vi "Send Light Message.vi"(9 "Lights":T1) -> (0 "error out":errorcluster)   [LabVIEW 2016]
uses:
  Light Reference.ctl
  <vilib>/Rock Robotics/WPI/SerialPort/WPI_SerialPortRef.ctl
  LED Send Global.vi
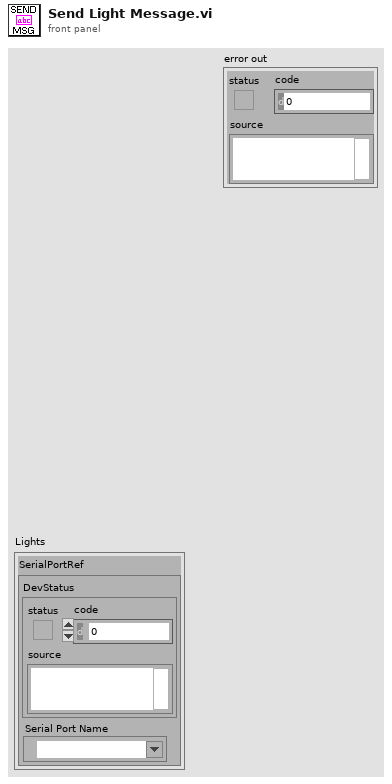
[diagram p1: front panel]
types:
  T1 = typedef "Light Reference.ctl" = cluster{"SerialPortRef":T2}
  T2 = typedef "WPI_SerialPortRef.ctl" = cluster{"DevStatus":errorcluster, "Serial Port Name":refnum<visa-resource-name>}
  T3 = typedef "LED Send Global.ctl" = cluster{"Underglow States":cluster{"RED":bool, "BLUE":bool}, "Hopper States":cluster{"No Shooter Power":bool, "1 RED":bool, "2 RED":bool, "3 RED":bool, "1 YEL 3 RED":bool, "2 YEL 3 RED":bool, "3 YEL 3 RED":bool, "1 GRN 3 YEL 3 RED":bool, "2 GRN 3 YEL 3 RED":bool, "3 GRN 3 YEL 3 RED":bool, "All GRN":bool, "Shooter w/Agitator":bool}, "License Plate States":cluster{"Auton States":cluster{"Do Nothing":bool, "Gear":bool, "Gear & Baseline":bool, "Gear & Shooter":bool, "Shooter":bool, "Shooter & Ball Dump":bool}, "Drive Train":cluster{"High Gear":bool, "Low Gear":bool}}, "Misc":cluster{"Pit/Demo":bool}, "Lights":cluster{"Underglow":string, "License Plate":string, "Hopper":string}}
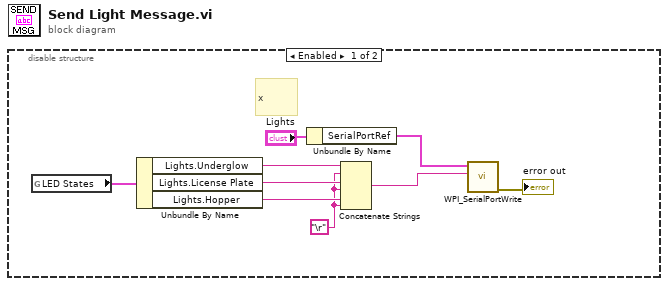
[diagram p0: block diagram]
diagram:
  n1 = disable-structure shown="Enabled" {
    frame Enabled {
      w5 = "\r"
      # "x"
      n2 = global read "LED Send Global.vi" "LED States"() -> (w3:T3)
      n3 = Unbundle By Name(w3) -> ("Lights.Underglow"=w9:string, "Lights.License Plate"=w6:string, "Lights.Hopper"=w7:string)
      n4 = Unbundle By Name("Lights") -> ("SerialPortRef"=w1:T2)
      n5 = Concatenate Strings(w9, w5, w6, w5, w7, w5) -> (w8:string)
      n6 = call <vilib>:"WPI_SerialPortWrite.vi"("Buffer"=w8, "SerialPortRef"=w1) -> ("error out"=→"error out":errorcluster)  [unwired: 7 in, 2 out]
    }
    frame Disabled {
    }
  }
